vi "Read or Write Systems Setup.vi"(0 "Base Setup In":T1, 5 "ServerPath":path, 7 "Write?":bool, 9 "Machine Type":string, 11 "Error In":errorcluster) -> (4 "Base Setup Out":T1, 15 "Error Out":errorcluster)   [LabVIEW 2013]
uses:
  <vilib>/Utility/config.llb/Read Key (String).vi
  <vilib>/Utility/config.llb/Write Key (String).vi
  <vilib>/Utility/config.llb/NI_LVConfig.lvlib
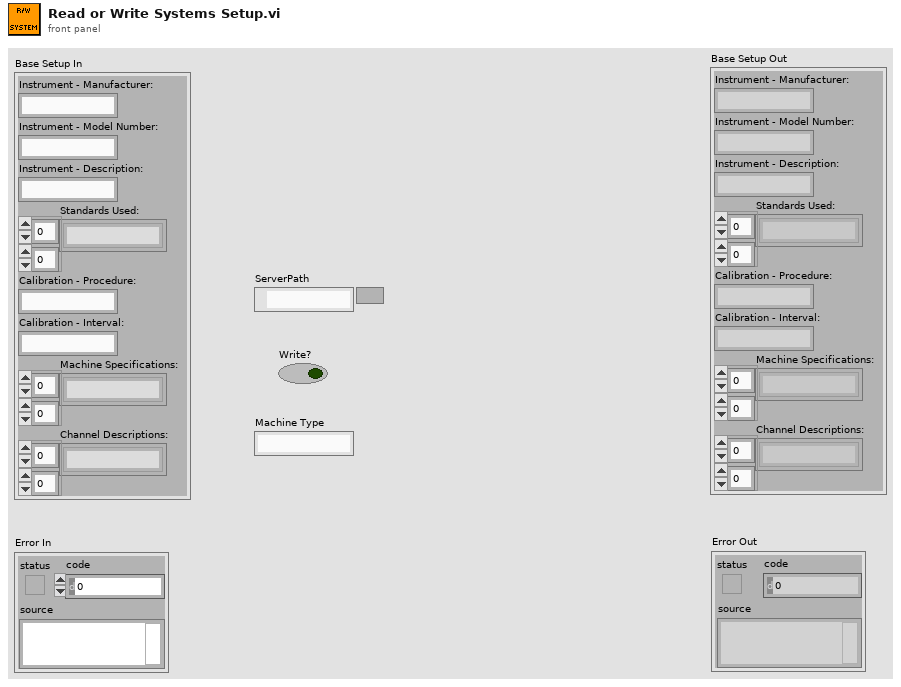
[diagram p1: front panel]
types:
  T1 = cluster{"Instrument - Manufacturer:":string, "Instrument - Model Number:":string, "Instrument - Description:":string, "Standards Used:":string[][], "Calibration - Procedure:":string, "Calibration - Interval:":string, "Machine Specifications:":string[][], "Channel Descriptions:":string[][]}
  T2 = typedef "NI_LVConfig.lvlib/Config Data RefNum.ctl" = refnum<k1>
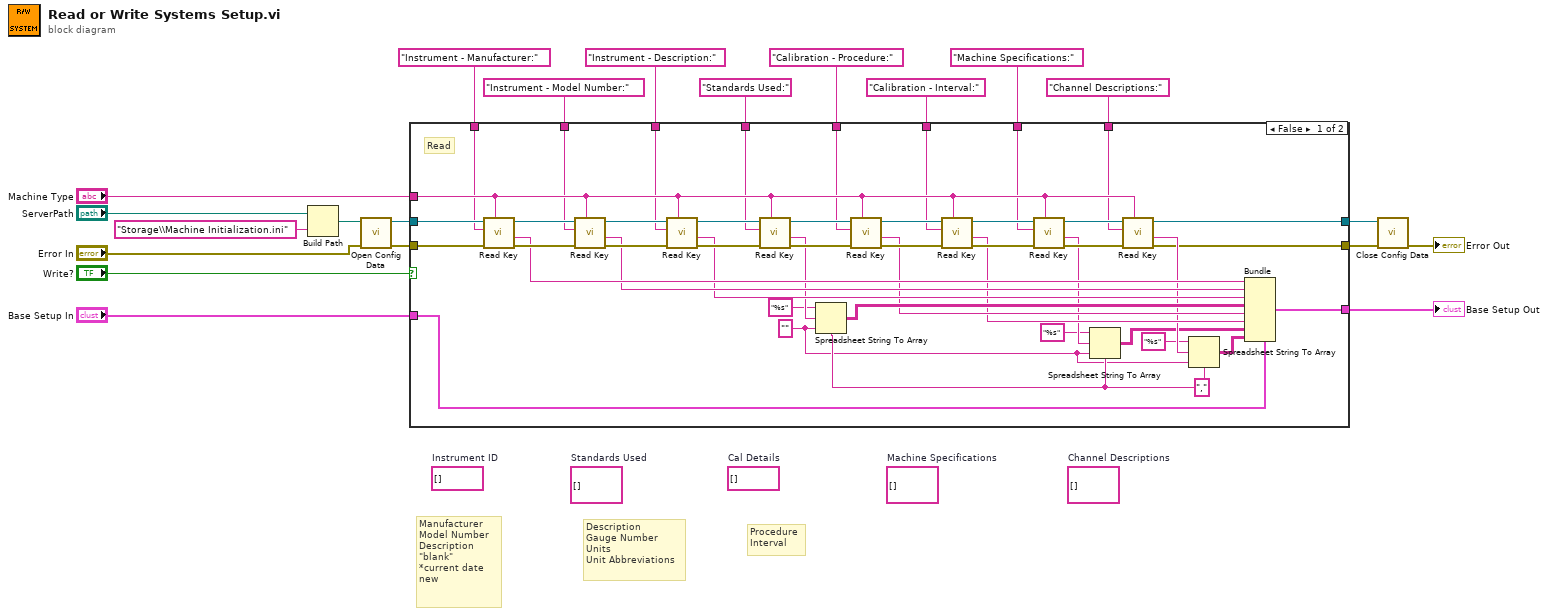
[diagram p0: block diagram]
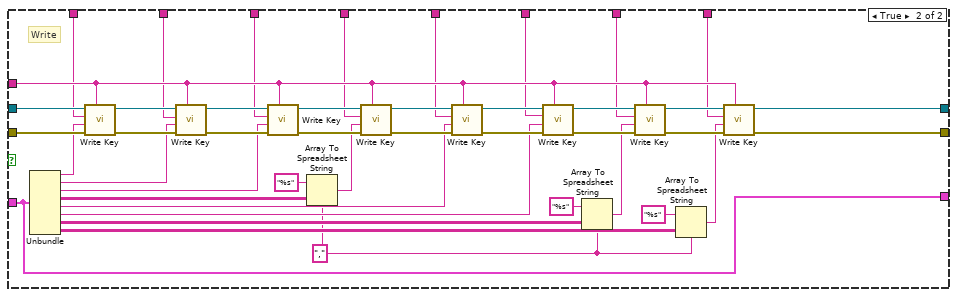
[diagram p2: hidden frame]
diagram:
  (unwired) string[][] []  # Channel Descriptions
  (unwired) string[][] []  # Machine Specifications
  (unwired) string[] []  # Cal Details
  (unwired) string[][] []  # Standards Used
  (unwired) string[] []  # Instrument ID
  # "Procedure\nInterval"
  # "Description\nGauge Number\nUnits\nUnit Abbreviations"
  # "Manufacturer\nModel Number\nDescription\n\"blank\"\n*current date\nnew"
  n1 = Build Path(base path="ServerPath", name or relative path="Storage\\Machine Initialization.ini") -> (appended path=w20:path)
  n2 = call <vilib>:"Open Config Data.vi"("error in (no error)"="Error In", "configuration file path"=w20) -> ("error out"=w14:errorcluster, "refnum"=w15:T2)  [unwired: 7 in, 1 out]
  n3 = case shown="False" "Write?" {
    tunnel: "Base Setup In" -> [w41 w70]
    tunnel: w15 -> [w66 w109]
    tunnel: w14 -> [w65 w108]
    tunnel: "Machine Type" -> [w50 w107]
    tunnel: "Instrument - Manufacturer:" -> [w42 w92]
    tunnel: "Instrument - Model Number:" -> [w43 w91]
    tunnel: "Instrument - Description:" -> [w44 w90]
    tunnel: "Standards Used:" -> [w45 w89]
    tunnel: "Calibration - Procedure:" -> [w46 w88]
    tunnel: "Calibration - Interval:" -> [w47 w87]
    tunnel: "Machine Specifications:" -> [w48 w86]
    tunnel: "Channel Descriptions:" -> [w49 w85]
    tunnel: [w26 w72] -> w1
    tunnel: [w27 w71] -> w2
    tunnel: [w25 w70] -> w4
    frame False {
      w29 = "," ("delimiter (Tab)")
      w28 = ""
      # "Read"
      n4 = call-poly <vilib>:"Read Key.vi"("section"=w50, "error in (no error)"=w65, "key"=w42, "refnum"=w66) -> ("error out"=w51:errorcluster, "value"=w40:string, "refnum out"=w64:T2)  [unwired: 4 in, 1 out]
      n5 = call-poly <vilib>:"Read Key.vi"("section"=w50, "error in (no error)"=w51, "key"=w43, "refnum"=w64) -> ("error out"=w52:errorcluster, "value"=w39:string, "refnum out"=w63:T2)  [unwired: 4 in, 1 out]
      n6 = call-poly <vilib>:"Read Key.vi"("section"=w50, "error in (no error)"=w52, "key"=w44, "refnum"=w63) -> ("error out"=w53:errorcluster, "value"=w38:string, "refnum out"=w62:T2)  [unwired: 4 in, 1 out]
      n7 = call-poly <vilib>:"Read Key.vi"("section"=w50, "error in (no error)"=w53, "key"=w45, "refnum"=w62) -> ("error out"=w54:errorcluster, "value"=w37:string, "refnum out"=w61:T2)  [unwired: 4 in, 1 out]
      n8 = Spreadsheet String To Array(delimiter (Tab)=w29, format string="%s", spreadsheet string=w37, array type (2D Dbl)=w28) -> (array=w36:string[][])
      n9 = call-poly <vilib>:"Read Key.vi"("section"=w50, "error in (no error)"=w54, "key"=w46, "refnum"=w61) -> ("error out"=w55:errorcluster, "value"=w35:string, "refnum out"=w60:T2)  [unwired: 4 in, 1 out]
      n10 = call-poly <vilib>:"Read Key.vi"("section"=w50, "error in (no error)"=w55, "key"=w47, "refnum"=w60) -> ("error out"=w56:errorcluster, "value"=w34:string, "refnum out"=w59:T2)  [unwired: 4 in, 1 out]
      n11 = call-poly <vilib>:"Read Key.vi"("section"=w50, "error in (no error)"=w56, "key"=w48, "refnum"=w59) -> ("error out"=w57:errorcluster, "value"=w33:string, "refnum out"=w58:T2)  [unwired: 4 in, 1 out]
      n12 = Spreadsheet String To Array(delimiter (Tab)=w29, format string="%s", spreadsheet string=w33, array type (2D Dbl)=w28) -> (array=w31:string[][])
      n13 = call-poly <vilib>:"Read Key.vi"("section"=w50, "error in (no error)"=w57, "key"=w49, "refnum"=w58) -> ("error out"=w26:errorcluster, "value"=w32:string, "refnum out"=w27:T2)  [unwired: 4 in, 1 out]
      n14 = Spreadsheet String To Array(delimiter (Tab)=w29, format string="%s", spreadsheet string=w32, array type (2D Dbl)=w28) -> (array=w30:string[][])
      n15 = Bundle(cluster=w41, "Instrument - Manufacturer:"=w40, "Instrument - Model Number:"=w39, "Instrument - Description:"=w38, "Standards Used:"=w36, "Calibration - Procedure:"=w35, "Calibration - Interval:"=w34, "Machine Specifications:"=w31, "Channel Descriptions:"=w30) -> (w25:T1)
    }
    frame True {
      w73 = "," ("delimiter (Tab)")
      # "Write"
      n16 = Unbundle(w70) -> ("Instrument - Manufacturer:"=w83:string, "Instrument - Model Number:"=w82:string, "Instrument - Description:"=w81:string, "Standards Used:"=w84:string[][], "Calibration - Procedure:"=w79:string, "Calibration - Interval:"=w78:string, "Machine Specifications:"=w77:string[][], "Channel Descriptions:"=w74:string[][])
      n17 = call-poly <vilib>:"Write Key.vi"("section"=w107, "error in (no error)"=w108, "value"=w83, "key"=w92, "refnum"=w109) -> ("error out"=w99:errorcluster, "refnum out"=w100:T2)  [unwired: 4 in, 1 out]
      n18 = call-poly <vilib>:"Write Key.vi"("section"=w107, "error in (no error)"=w99, "value"=w82, "key"=w91, "refnum"=w100) -> ("error out"=w98:errorcluster, "refnum out"=w101:T2)  [unwired: 4 in, 1 out]
      n19 = call-poly <vilib>:"Write Key.vi"("section"=w107, "error in (no error)"=w98, "value"=w81, "key"=w90, "refnum"=w101) -> ("error out"=w97:errorcluster, "refnum out"=w102:T2)  [unwired: 4 in, 1 out]
      n20 = Array To Spreadsheet String(delimiter (Tab)=w73, array=w84, 3:"%s" ("format string")) -> (spreadsheet string=w80:string)
      n21 = call-poly <vilib>:"Write Key.vi"("section"=w107, "error in (no error)"=w97, "value"=w80, "key"=w89, "refnum"=w102) -> ("error out"=w96:errorcluster, "refnum out"=w103:T2)  [unwired: 4 in, 1 out]
      n22 = call-poly <vilib>:"Write Key.vi"("section"=w107, "error in (no error)"=w96, "value"=w79, "key"=w88, "refnum"=w103) -> ("error out"=w95:errorcluster, "refnum out"=w104:T2)  [unwired: 4 in, 1 out]
      n23 = call-poly <vilib>:"Write Key.vi"("section"=w107, "error in (no error)"=w95, "value"=w78, "key"=w87, "refnum"=w104) -> ("error out"=w94:errorcluster, "refnum out"=w105:T2)  [unwired: 4 in, 1 out]
      n24 = Array To Spreadsheet String(delimiter (Tab)=w73, array=w77, 3:"%s" ("format string")) -> (spreadsheet string=w76:string)
      n25 = call-poly <vilib>:"Write Key.vi"("section"=w107, "error in (no error)"=w94, "value"=w76, "key"=w86, "refnum"=w105) -> ("error out"=w93:errorcluster, "refnum out"=w106:T2)  [unwired: 4 in, 1 out]
      n26 = Array To Spreadsheet String(delimiter (Tab)=w73, array=w74, 3:"%s" ("format string")) -> (spreadsheet string=w75:string)
      n27 = call-poly <vilib>:"Write Key.vi"("section"=w107, "error in (no error)"=w93, "value"=w75, "key"=w85, "refnum"=w106) -> ("error out"=w72:errorcluster, "refnum out"=w71:T2)  [unwired: 4 in, 1 out]
    }
  }
  "Base Setup Out" <- w4
  n28 = call <vilib>:"Close Config Data.vi"("error in (no error)"=w1, "refnum"=w2) -> ("error out"=→"Error Out":errorcluster)  [unwired: 8 in, 1 out]
